vi "Untitled 5.vi"() -> ()   [LabVIEW 2023, in "Driver.lvlib"]
uses:
  Driver.lvlib
  Driver/Driver.lvclass
panel:
  out "Version":string
  out "Error buffer":string
  out "ID_DEVICE":string
  out "error out":errorcluster
  in  "error in (no error)":errorcluster
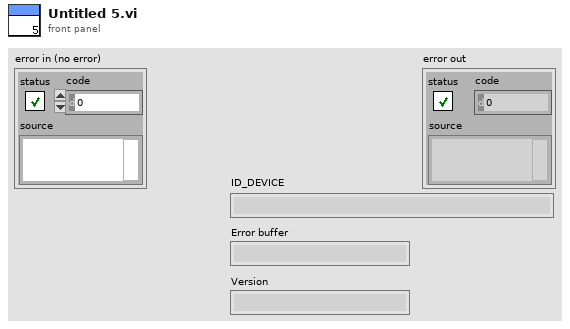
[diagram p1: front panel]
types:
  T1 = cluster{"VISA Refnum":refnum<visa-resource-name>, "Baud Rate":u32, "Timeout":u32}
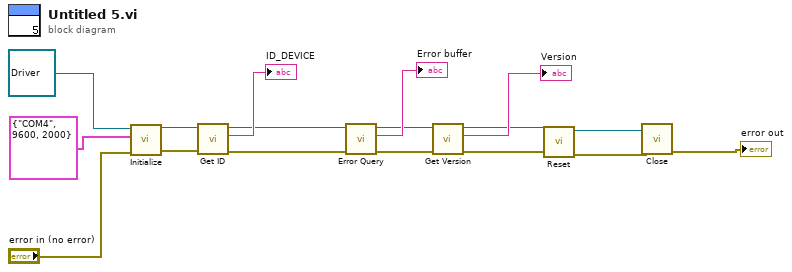
[diagram p0: block diagram]
diagram:
  n1 = call-dynamic "Initialize.vi"("error in (no error)"="error in (no error)", "Input"=T1 {"VISA Refnum"="COM4", "Baud Rate"=9600, "Timeout"=2000}, "Driver in"=refnum<class "Driver.lvclass"> refnum) -> ("error out"=w14:errorcluster, "Driver out"=w13:refnum<class "Driver.lvclass">)  [unwired: 7 in]
  n2 = call-dynamic "Get ID.vi"("error in (no error)"=w14, "Driver in"=w13) -> ("error out"=w9:errorcluster, "ID_DEVICE"=→"ID_DEVICE":string, "Driver out"=w10:refnum<class "Driver.lvclass">)  [unwired: 7 in]
  n3 = call-dynamic "Error Query.vi"("error in (no error)"=w9, "Driver in"=w10) -> ("error out"=w6:errorcluster, "read buffer"=→"Error buffer":string, "Driver out"=w7:refnum<class "Driver.lvclass">)  [unwired: 7 in]
  n4 = call-dynamic "Get Version.vi"("error in (no error)"=w6, "Driver in"=w7) -> ("error out"=w1:errorcluster, "Version"=→"Version":string, "Driver out"=w2:refnum<class "Driver.lvclass">)  [unwired: 7 in]
  n5 = call-dynamic "Reset.vi"("error in (no error)"=w1, "Driver in"=w2) -> ("error out"=w4:errorcluster, "Driver out"=w3:refnum<class "Driver.lvclass">)  [unwired: 8 in]
  n6 = call-dynamic "Close.vi"("error in (no error)"=w4, "Driver in"=w3) -> ("error out"=→"error out":errorcluster)  [unwired: 8 in, 1 out]
